vi "BB_Check_Camera_IP_Change.vi"(8 "error in":errorcluster, 9 "Camera Settings In":T1={"Frate Rate"=30, "Compression"=30, "Size"=1} {"Frate Rate" scale=1.0..30.0; "Size" items=["640x480", "320x240", "160x120"]}, 10 "Image In":T2, 11 "Incoming IP":string) -> (0 "error out":errorcluster, 1 "Camera Settings Out":T1={"Frate Rate"=30, "Compression"=30, "Size"=1} {"Frate Rate" scale=1.0..30.0; "Size" items=["640x480", "320x240", "160x120"]}, 2 "Image Out":T2, 3 "IP Out":string="IP Out")   [LabVIEW 2012]
uses:
  <vilib>/vision/Image Controls.llb/IMAQ Image.ctl
panel:
  in  "Last IP":i32
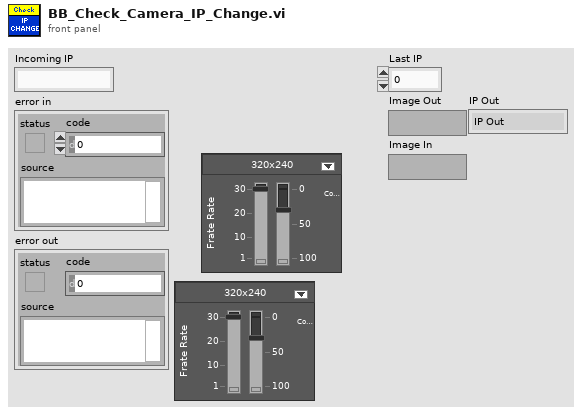
[diagram p1: front panel]
types:
  T1 = cluster{"Frate Rate":i32, "Compression":i32, "Size":u16}
  T2 = typedef "IMAQ Image.ctl" = refnum<image>
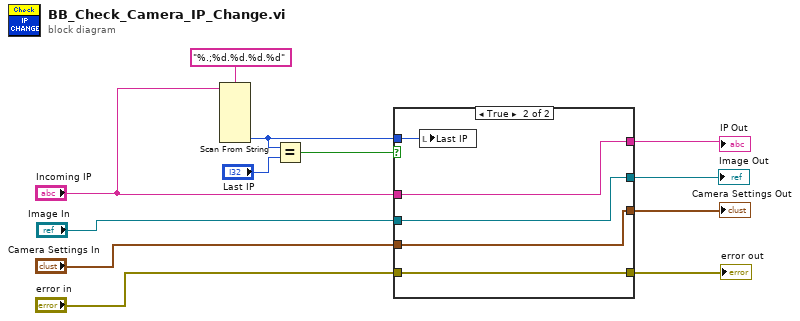
[diagram p0: block diagram]
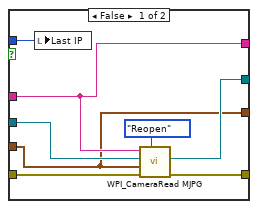
[diagram p2: hidden frame]
diagram:
  n1 = Scan From String(format string="%.;%d.%d.%d.%d", input string="Incoming IP") -> (output 4=w7:i32)  [unwired: 2 in, 10 out]
  n2 = Equal?(x=w7, y="Last IP") -> (x = y?=w11:bool)
  n3 = case shown="True" w11 {
    tunnel: w7 -> [w20 w25]
    tunnel: "Camera Settings In" -> [w13 w21]
    tunnel: "Incoming IP" -> [w14 w22]
    tunnel: "error in" -> [w18 w24]
    tunnel: [w17 w24] -> w3
    tunnel: [w16 w23] -> w4
    tunnel: "Image In" -> [w15 w23]
    tunnel: [w14 w22] -> w2
    tunnel: [w13 w21] -> w1
    frame False {
      n4 = local write "Last IP"(w20) -> ()
      n5 = call <vilib>:"WPI_CameraRead MJPG.vi"("Operation"=enum16{"Read", "Reopen", "Close"}."Reopen", "error in"=w18, "Camera Settings"=w13, "Image"=w15, "address"=w14) -> ("error out"=w17:errorcluster, "Image Out"=w16:T2)  [unwired: 4 in, 1 out]
    }
    frame True {
      n6 = local write "Last IP"(w25) -> ()
    }
  }
  "Image Out" <- w4
  "error out" <- w3
  "IP Out" <- w2
  "Camera Settings Out" <- w1
